vi "decode_p11.vi"(11 "file path (dialog if empty)":path) -> (1 "HeadeR":string[](array[string]), 2 "Data":string[](array[string]), 3 "all rows":string[][](array[string]))   [LabVIEW 2020]
uses:
  <vilib>/Utility/file.llb/Read Delimited Spreadsheet (string).vi
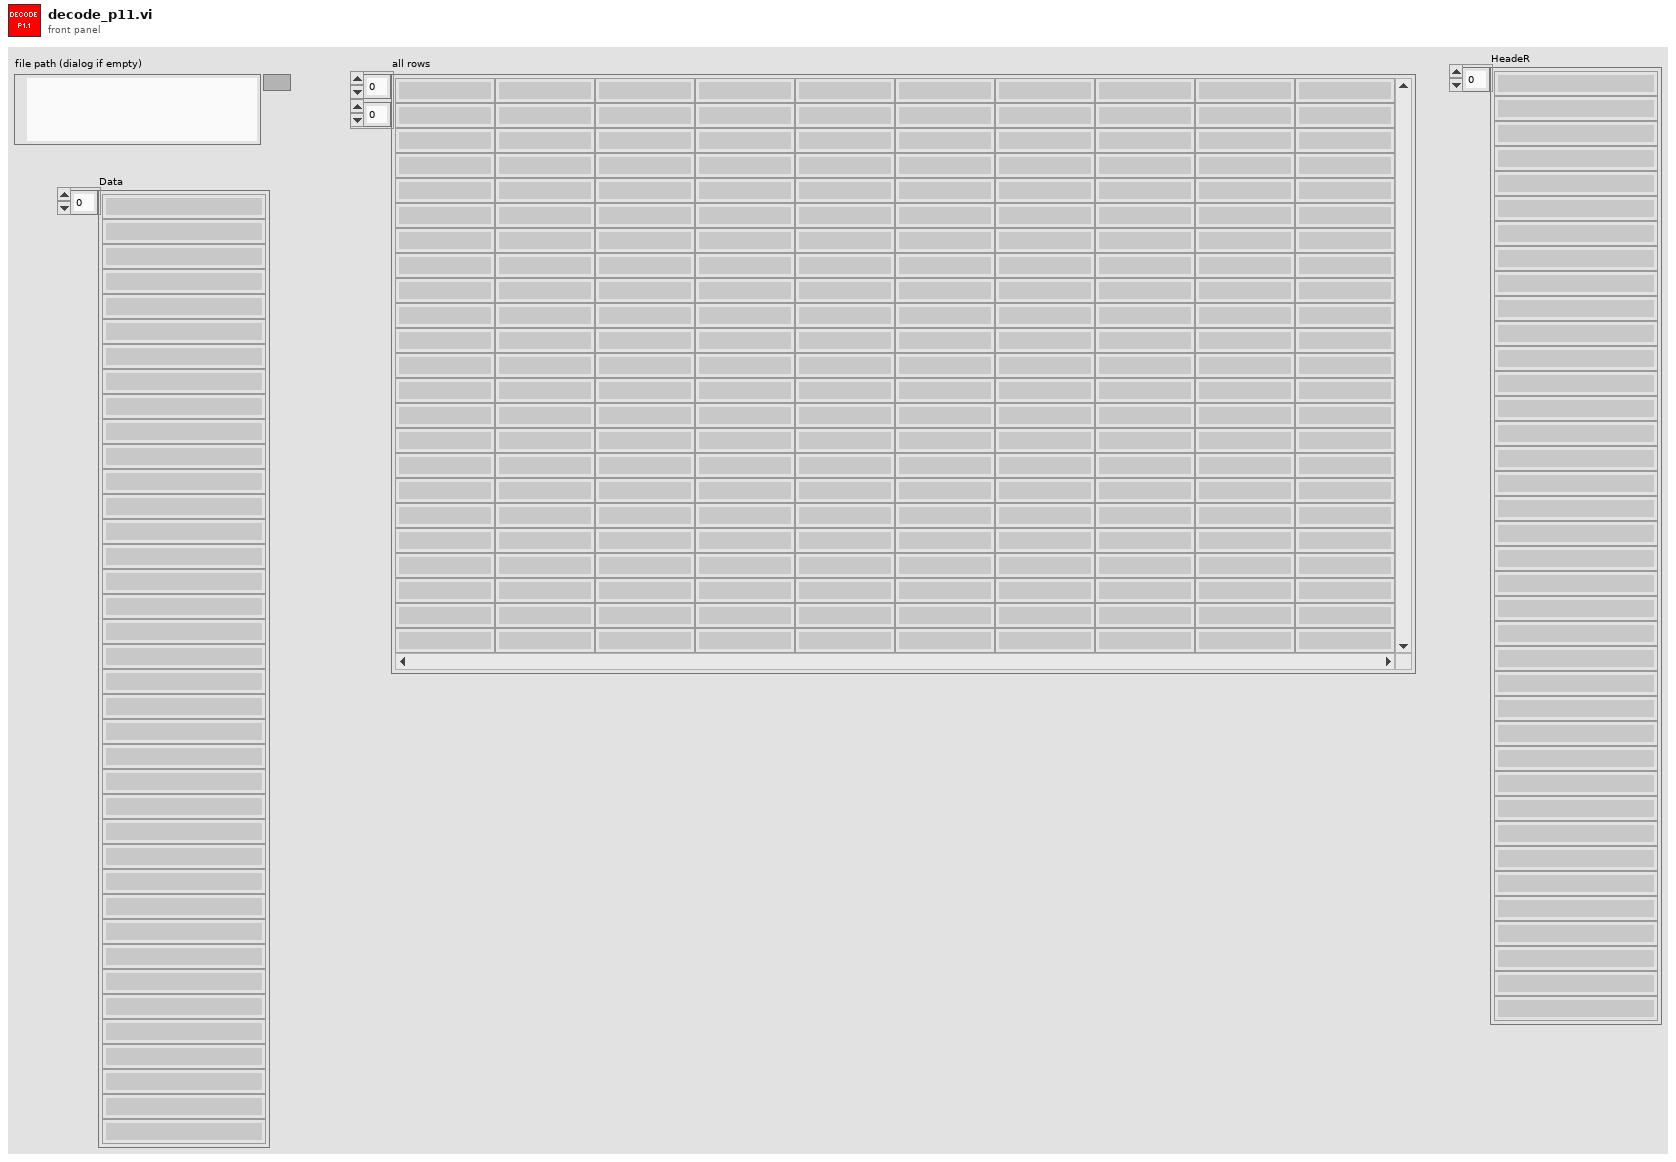
[diagram p1: front panel]
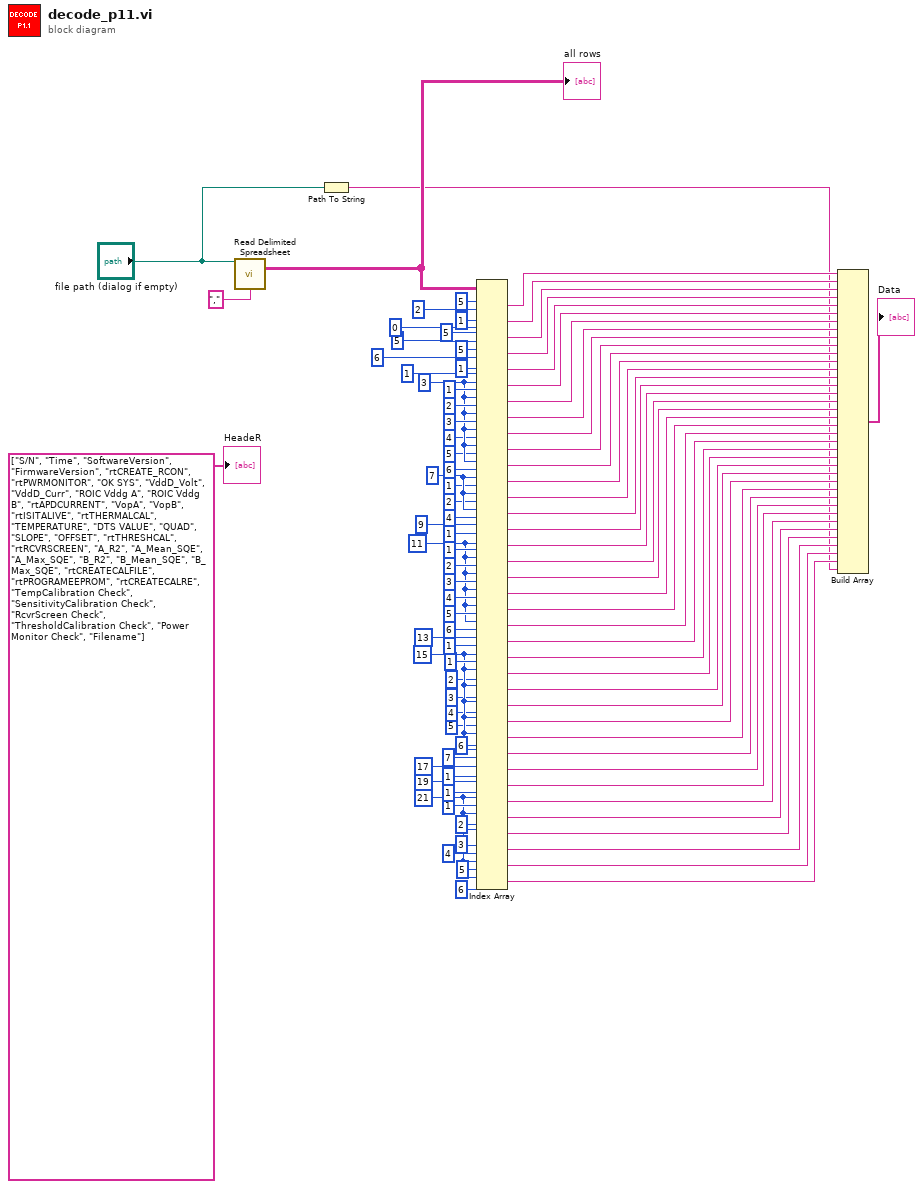
[diagram p0: block diagram]
diagram:
  w17 = 21 ("disabled index (row)")
  w36 = 15 ("index (row)")
  w48 = 11 ("disabled index (row)")
  w63 = 7 ("index (row)")
  w72 = 3 ("index (row)")
  n1 = call-poly <vilib>:"Read Delimited Spreadsheet.vi"("file path (dialog if empty)"="file path (dialog if empty)", "delimiter (\\t)"="," ("delimiter (\\t)")) -> ("all rows"=w93:string[][])  [unwired: 8 in, 5 out]
  "all rows" <- w93
  n2 = Path To String(path="file path (dialog if empty)") -> (string=w1:string)
  n3 = Index Array(array=w93, index (row) #1=5 ("index (row)"), index (col) #1=2 ("disabled index (col)"), index (row) #2=1 ("index (row)"), index (col) #2=0 ("disabled index (col)"), index (row) #3=5 ("index (row)"), index (col) #3=5 ("disabled index (col)"), index (row) #4=5 ("index (row)"), index (col) #4=6 ("disabled index (col)"), index (row) #5=1 ("index (row)"), index (col) #5=1 ("disabled index (col)"), index (row) #6=w72, index (col) #6=1 ("disabled index (col)"), index (row) #7=w72, index (col) #7=2 ("disabled index (col)"), index (row) #8=w72, index (col) #8=3 ("disabled index (col)"), index (row) #9=w72, index (col) #9=4 ("disabled index (col)"), index (row) #10=w72, index (col) #10=5 ("disabled index (col)"), index (row) #11=w72, index (col) #11=6 ("disabled index (col)"), index (row) #12=w63, index (col) #12=1 ("disabled index (col)"), index (row) #13=w63, index (col) #13=2 ("disabled index (col)"), index (row) #14=w63, index (col) #14=4 ("disabled index (col)"), index (row) #15=9 ("disabled index (row)"), index (col) #15=1 ("index (col)"), index (row) #16=w48, index (col) #16=1 ("index (col)"), index (row) #17=w48, index (col) #17=2 ("disabled index (col)"), index (row) #18=w48, index (col) #18=3 ("index (col)"), index (row) #19=w48, index (col) #19=4 ("index (col)"), index (row) #20=w48, index (col) #20=5 ("index (col)"), index (row) #21=w48, index (col) #21=6 ("disabled index (col)"), index (row) #22=13 ("disabled index (row)"), index (col) #22=1 ("index (col)"), index (row) #23=w36, index (col) #23=1 ("disabled index (col)"), index (row) #24=w36, index (col) #24=2 ("disabled index (col)"), index (row) #25=w36, index (col) #25=3 ("disabled index (col)"), index (row) #26=w36, index (col) #26=4 ("disabled index (col)"), index (row) #27=w36, index (col) #27=5 ("disabled index (col)"), index (row) #28=w36, index (col) #28=6 ("disabled index (col)"), index (row) #29=w36, index (col) #29=7 ("disabled index (col)"), index (row) #30=17 ("index (row)"), index (col) #30=1 ("disabled index (col)"), index (row) #31=19 ("disabled index (row)"), index (col) #31=1 ("index (col)"), index (row) #32=w17, index (col) #32=1 ("index (col)"), index (row) #33=w17, index (col) #33=2 ("disabled index (col)"), index (row) #34=w17, index (col) #34=3 ("disabled index (col)"), index (row) #35=w17, index (col) #35=4 ("disabled index (col)"), index (row) #36=w17, index (col) #36=5 ("disabled index (col)"), index (row) #37=w17, index (col) #37=6 ("disabled index (col)")) -> (element #1=w89:string, element #2=w86:string, element #3=w83:string, element #4=w80:string, element #5=w76:string, element #6=w75:string, element #7=w68:string, element #8=w67:string, element #9=w66:string, element #10=w65:string, element #11=w64:string, element #12=w59:string, element #13=w58:string, element #14=w57:string, element #15=w47:string, element #16=w46:string, element #17=w45:string, element #18=w44:string, element #19=w43:string, element #20=w42:string, element #21=w41:string, element #22=w38:string, element #23=w29:string, element #24=w28:string, element #25=w27:string, element #26=w26:string, element #27=w25:string, element #28=w24:string, element #29=w23:string, element #30=w11:string, element #31=w10:string, element #32=w9:string, element #33=w8:string, element #34=w7:string, element #35=w6:string, element #36=w5:string, element #37=w4:string)
  n4 = Build Array(w89, w86, w83, w80, w76, w75, w68, w67, w66, w65, w64, w59, w58, w57, w47, w46, w45, w44, w43, w42, w41, w38, w29, w28, w27, w26, w25, w24, w23, w11, w10, w9, w8, w7, w6, w5, w4, w1) -> (→"Data":string[])
  "HeadeR" <- string[] ["S/N", "Time", "SoftwareVersion", "FirmwareVersion", "rtCREATE_RCON", "rtPWRMONITOR", "OK SYS", "VddD_Volt", "VddD_Curr", "ROIC Vddg A", "ROIC Vddg B", "rtAPDCURRENT", "VopA", "VopB", "rtISITALIVE", "rtTHERMALCAL", "TEMPERATURE", "DTS VALUE", "QUAD", "SLOPE", "OFFSET", "rtTHRESHCAL", "rtRCVRSCREEN", "A_R2", "A_Mean_SQE", "A_Max_SQE", "B_R2", "B_Mean_SQE", "B_Max_SQE", "rtCREATECALFILE", "rtPROGRAMEEPROM", "rtCREATECALRE", "TempCalibration Check", "SensitivityCalibration Check", "RcvrScreen Check", "ThresholdCalibration Check", "Power Monitor Check", "Filename"] ("appended array 2")
